vi "SSH Set Pipe Descriptor.vi"(8 "Error In":errorcluster, 10 "SSH Pipe Descriptor":i32=-1, 11 "SSH Session":refnum<k1>) -> (0 "Error Out":errorcluster, 3 "SSH Session":refnum<k1>)   [LabVIEW 2019, in "LMH-LINX.lvlib"]
uses:
  <vilib>/MakerHub/LINX/LMH-LINX.lvlib
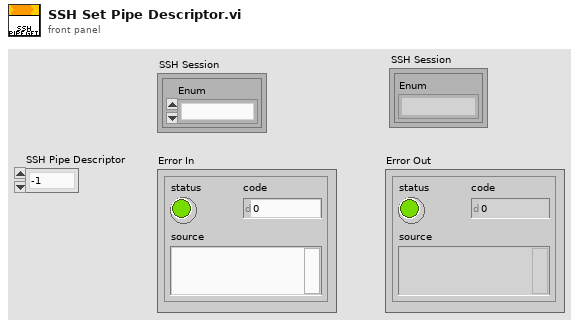
[diagram p1: front panel]
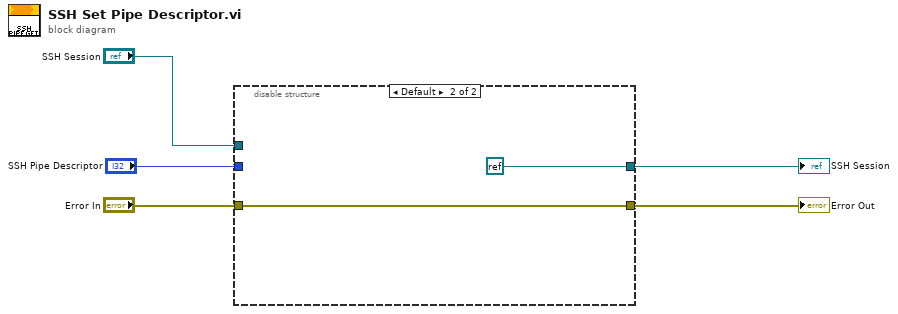
[diagram p0: block diagram]
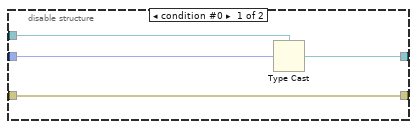
[diagram p2: hidden frame]
diagram:
  n1 = disable-structure shown="Default" {
    disable-tunnel: [w8 w11] -> w4
    disable-tunnel: "Error In" -> [w8 w11]
    disable-tunnel: "SSH Pipe Descriptor" -> [w9 _]
    disable-tunnel: [w7 refnum<k0> refnum] -> w1
    disable-tunnel: "SSH Session" -> [w6 _]
    frame condition #0 {
      n2 = Type Cast(type=w6, x=w9) -> (*(type *) &x=w7:refnum<k1>)
    }
    frame condition #1 (active) {
    }
  }
  "Error Out" <- w4
  "SSH Session" <- w1
